vi "Get Rove Header.vi"(8 "error in (no error)":errorcluster, 11 "TTLControl in":refnum<class "TTLController.lvclass">) -> (0 "error out":errorcluster, 2 "FileString":string[](array[string]), 3 "TTLControl out":refnum<class "TTLController.lvclass">)   [LabVIEW 2020, in "TTLController.lvclass"]
uses:
  TTLController.lvclass
  TTLController.lvclass/TTLController.ctl
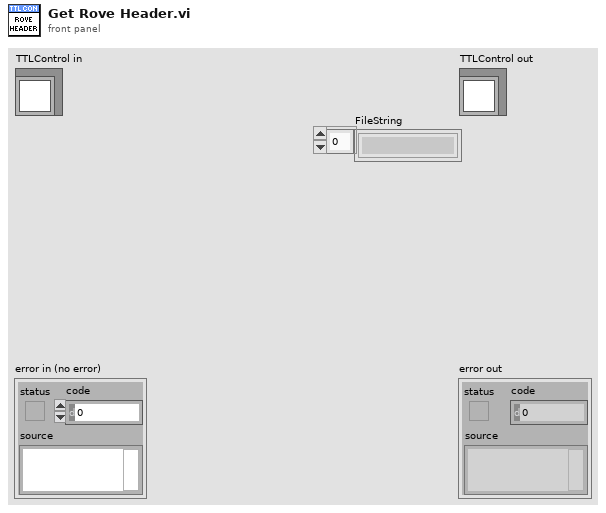
[diagram p1: front panel]
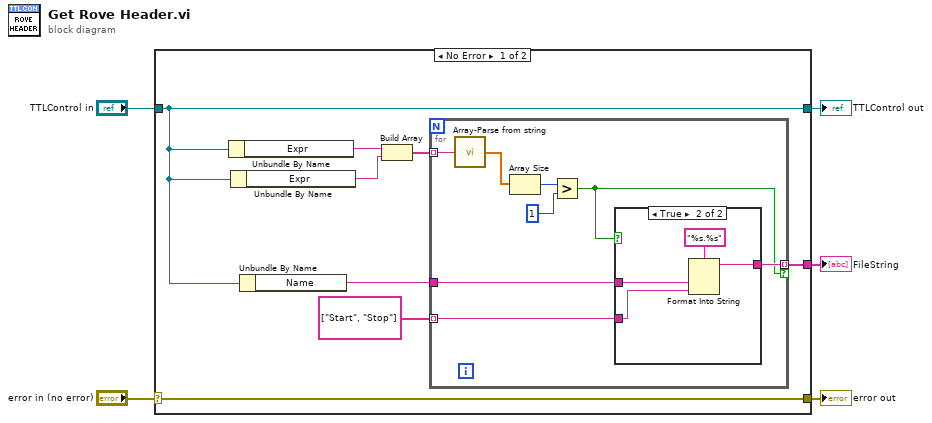
[diagram p0: block diagram]
diagram:
  n1 = case shown="No Error" "error in (no error)" {
    selector: "error in (no error)" -> [w13 w27]
    tunnel: [w13 w27] -> w4
    tunnel: [w11 w26] -> w2
    tunnel: "TTLControl in" -> [w11 w26]
    tunnel: [w6 _] -> w1
    frame No Error {
      n2 = Unbundle By Name(w11) -> ("Expr"=w12:string)
      n3 = Unbundle By Name(w11) -> ("Expr"=w8:string)
      n4 = Unbundle By Name(w11) -> ("Name"=w10:string)
      n5 = Build Array(w12, w8) -> (w9:string[])
      n6 = for {
        tunnel: w9 -> [w21] mode=indexing
        tunnel: w10 -> [w18]
        tunnel: string[] ["Start", "Stop"] -> [w17] mode=indexing
        tunnel: [w16] -> w6 mode=indexing if=w15
        n7 = call "Array-Parse from string.vi"("String"=w21) -> ("Array"=w20:dbl[])  [unwired: 13 in, 1 out]
        n8 = Array Size(array=w20) -> (size(s)=w19:i32)
        n9 = Greater?(x=w19, y=1) -> (0:w15:bool)
        n10 = case shown="True" w15 {
          tunnel: w18 -> [_ w24]
          tunnel: w17 -> [_ w23]
          tunnel: [_ w22] -> w16
          frame False {
          }
          frame True {
            n11 = Format Into String(format string="%s.%s", w24, w23) -> (resulting string=w22:string)  [unwired: 2 in, 1 out]
          }
        }
      }
    }
    frame Error {
    }
  }
  "error out" <- w4
  "TTLControl out" <- w2
  "FileString" <- w1
